vi "ClassifyRX.vi"(8 "error in (no error)":errorcluster, 10 "msg to Log":string, 11 "Log in":refnum<class "Log.lvclass">) -> (0 "error out":errorcluster, 3 "Log out":refnum<class "Log.lvclass">)   [LabVIEW 2018, in "Log.lvclass"]
uses:
  Log.lvclass
  Log.lvclass/Log.ctl
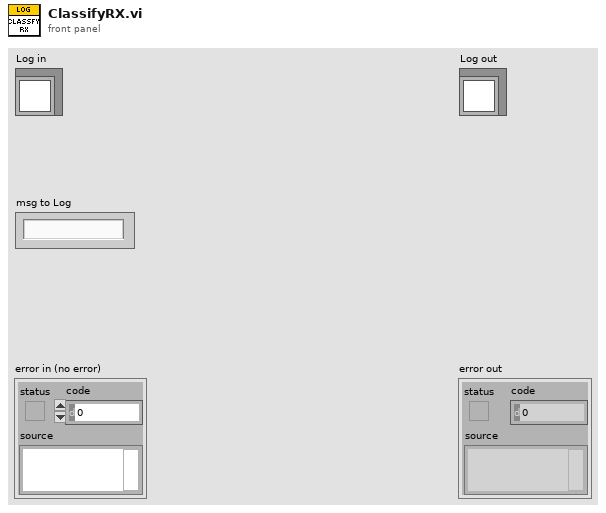
[diagram p1: front panel]
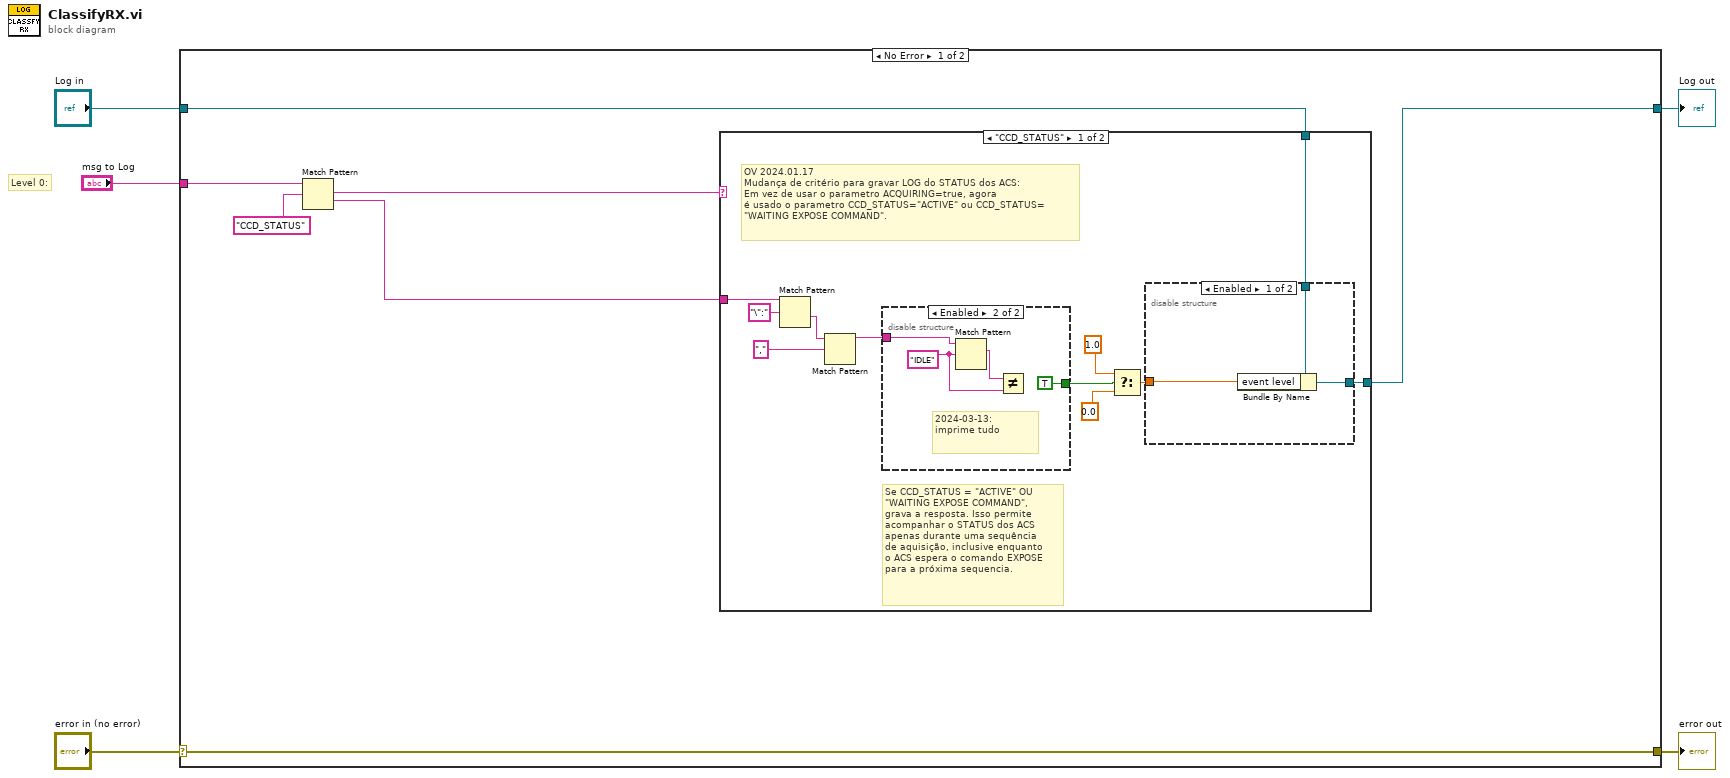
[diagram p0: block diagram]
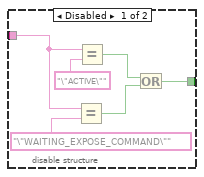
[diagram p2: hidden frame]
diagram:
  # "Level 0:"
  n1 = case shown="No Error" "error in (no error)" {
    selector: "error in (no error)" -> [w12 w40]
    tunnel: [w12 w40] -> w4
    tunnel: [w8 w39] -> w2
    tunnel: "Log in" -> [w9 w39]
    tunnel: "msg to Log" -> [w10 _]
    frame No Error {
      n2 = Match Pattern(string=w10, regular expression="CCD_STATUS") -> (match substring=w7:string, after substring=w6:string)  [unwired: 1 in, 2 out]
      n3 = case shown="\"CCD_STATUS\"" w7 {
        tunnel: w9 -> [w23 w38]
        tunnel: [w22 w38] -> w8
        tunnel: w6 -> [w21 _]
        frame "CCD_STATUS" {
          # "OV 2024.01.17\nMudança de critério para gravar LOG do STATUS dos ACS:\nEm vez de usar o parametro ACQUIRING=true, agora\né usado o parametro CCD_STATUS=\"ACTIVE\" ou CCD_STATUS=\n\"WAITING EXPOSE COMMAND\"."
          # "Se CCD_STATUS = \"ACTIVE\" OU \n\"WAITING EXPOSE COMMAND\", \ngrava a resposta. Isso permite \nacompanhar o STATUS dos ACS \napenas durante uma sequência \nde aquisição, inclusive enquanto \no ACS espera o comando EXPOSE\npara a próxima sequencia."
          n4 = Match Pattern(string=w21, regular expression="\":") -> (after substring=w19:string)  [unwired: 1 in, 3 out]
          n5 = Match Pattern(string=w19, regular expression=",") -> (before substring=w15:string)  [unwired: 1 in, 3 out]
          n6 = disable-structure shown="Enabled" {
            disable-tunnel: [w25 TRUE] -> w16
            disable-tunnel: w15 -> [w24 w33]
            frame Disabled {
              n7 = Equal?(x=w24, y="\"WAITING_EXPOSE_COMMAND\"") -> (x = y?=w26:bool)
              n8 = Equal?(x=w24, y="\"ACTIVE\"") -> (x = y?=w27:bool)
              n9 = Or(x=w27, y=w26) -> (x .or. y?=w25:bool)
            }
            frame Enabled {
              w31 = "IDLE"
              # "2024-03-13:\nimprime tudo"
              n10 = Match Pattern(string=w33, regular expression=w31) -> (match substring=w32:string)  [unwired: 1 in, 3 out]
              n11 = Not Equal?(x=w32, y=w31) -> ()  [unwired: 1 out]
            }
          }
          n12 = Select(t=1.0 ("current level"), s=w16, f=0.0) -> (s? t:f=w17:dbl)
          n13 = disable-structure shown="Enabled" {
            disable-tunnel: w23 -> [w36 w37]
            disable-tunnel: [w35 w37] -> w22
            disable-tunnel: w17 -> [w34 _]
            frame Enabled {
              n14 = Bundle By Name(cluster=w36, "event level"=w34) -> (w35:refnum<class "Log.lvclass">)
            }
            frame Disabled {
            }
          }
        }
        frame Default {
        }
      }
    }
    frame Error {
    }
  }
  "error out" <- w4
  "Log out" <- w2
